vi "SetSpeed1.vi"(11 "Chaîne":string) -> ()   [LabVIEW 2015]
panel:
  in  "error in (no error) 2":errorcluster
  out "error in (no error)":errorcluster
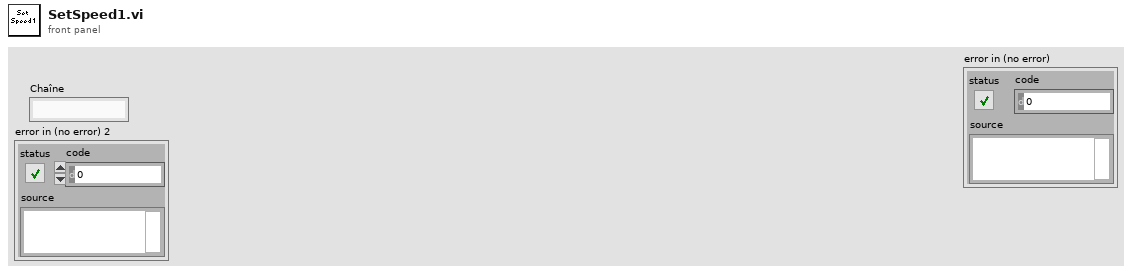
[diagram p1: front panel]
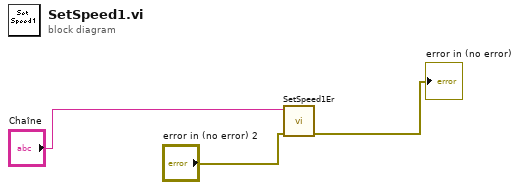
[diagram p0: block diagram]
diagram:
  n1 = call "SetSpeed1Er.vi"("error in (no error)"="error in (no error) 2", "Chaîne"="Chaîne") -> ("error out"=→"error in (no error)":errorcluster)  [unwired: 9 in]
